vi "Encode (Single Param).vi"(9 "parameter in":dbl, 10 "parameter configuration":T1, 11 "words in":u16[](array[numeric]) format="%.0b") -> (3 "words out":u16[](array[numeric]) format="%.0b")   [LabVIEW 2020]
uses:
  _typedefs/parameter_config_type.ctl
  _typedefs/parameter_config_type_type.ctl
  _typedefs/parameter_config_encoding_type.ctl
  datatypes/dt_encodeDecode.lvlib
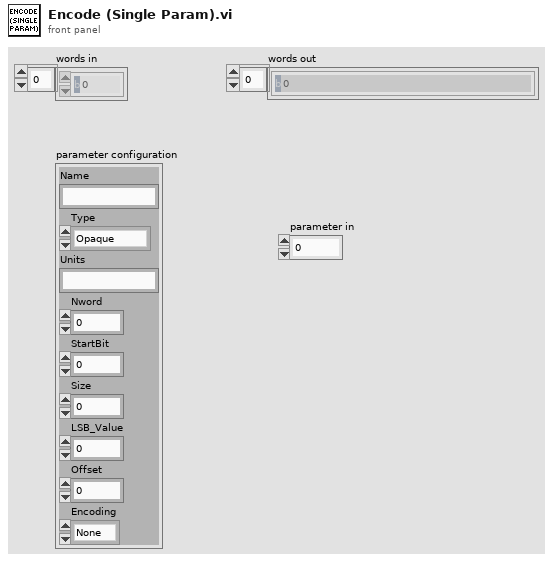
[diagram p1: front panel]
types:
  T1 = typedef "parameter_config_type.ctl" = cluster{"Name":string, "Type":T2, "Units":string, "Nword":i32, "StartBit":i32, "Size":i32, "LSB_Value":dbl, "Offset":i32, "Encoding":T3}
  T2 = typedef "parameter_config_type_type.ctl" = enum16{"Opaque", "Enum", "Float", "Integer", "Bcd", "Bool"}
  T3 = typedef "parameter_config_encoding_type.ctl" = enum16{"None", "2-complement", "Unsigned"}
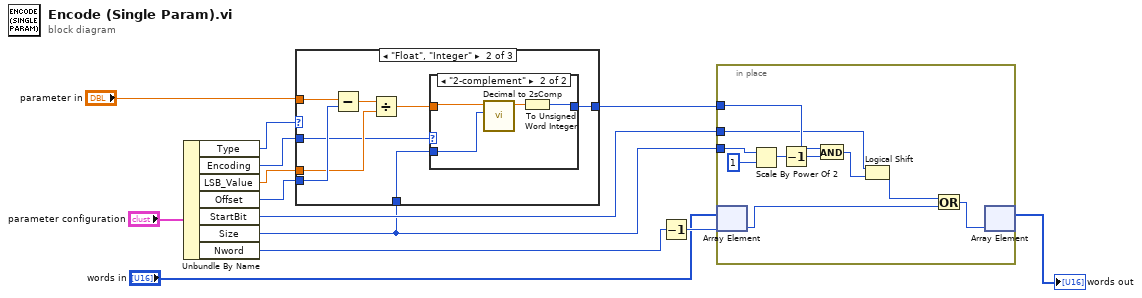
[diagram p0: block diagram]
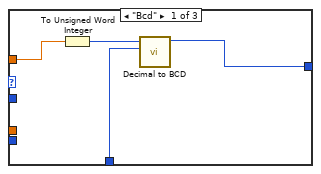
[diagram p2: hidden frame]
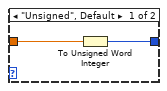
[diagram p3: hidden frame]
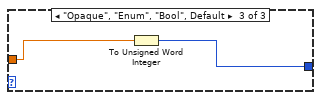
[diagram p4: hidden frame]
diagram:
  n1 = Unbundle By Name("parameter configuration") -> ("Type"=w6:T2, "Encoding"=w4:T3, "LSB_Value"=w3:dbl, "Offset"=w2:i32, "StartBit"=w12:i32, "Size"=w5:i32, "Nword"=w8:i32)
  n2 = case shown="\"Float\", \"Integer\"" w6 {
    tunnel: "parameter in" -> [w17 w25 w33]
    tunnel: w5 -> [w16 w18 _]
    tunnel: w4 -> [_ w21 _]
    tunnel: w3 -> [_ w22 _]
    tunnel: w2 -> [_ w24 _]
    tunnel: [w15 w19 w32] -> w1
    frame "Bcd" {
      n3 = To Unsigned Word Integer(number=w17) -> (unsigned 16bit integer=w14:u16)
      n4 = call "Decimal to BCD.vi"("size in bits"=w16, "decimal data in"=w14) -> ("bcd data out"=w15:u16)  [unwired: 9 in]
    }
    frame "Float", "Integer" {
      n5 = Subtract(x=w25, y=w24) -> (x-y=w23:dbl)
      n6 = Divide(x=w23, y=w22) -> (x/y=w20:dbl)
      n7 = case shown="\"2-complement\"" w21 {
        tunnel: w20 -> [w27 w30]
        tunnel: [w26 w28] -> w19
        tunnel: w18 -> [_ w31]
        frame "Unsigned", Default {
          n8 = To Unsigned Word Integer(number=w27) -> (unsigned 16bit integer=w26:u16)
        }
        frame "2-complement" {
          n9 = call "Decimal to 2sComp.vi"("size in bit"=w31, "decimal in"=w30) -> ("word out"=w29:dbl)  [unwired: 9 in]
          n10 = To Unsigned Word Integer(number=w29) -> (unsigned 16bit integer=w28:u16)
        }
      }
    }
    frame "Opaque", "Enum", "Bool", Default {
      n11 = To Unsigned Word Integer(number=w33) -> (unsigned 16bit integer=w32:u16)
    }
  }
  n12 = Decrement(x=w8) -> (x-1=w11:i32)
  n13 = in-place {
    in-place-border: w5 -> [w42]
    in-place-border: w1 -> [w39]
    in-place-border: w12 -> [w38]
    n14 = in-place-array #1("words in", w11) -> (w35:u16)
    n15 = Scale By Power Of 2(n=w42, x=u16 1) -> (x*2^n=w41:u16)
    n16 = Decrement(x=w41) -> (x-1=w40:u16)
    n17 = And(x=w39, y=w40) -> (x .and. y?=w37:u16)
    n18 = Logical Shift(y=w38, x=w37) -> (x << y=w36:u16)
    n19 = Or(x=w36, y=w35) -> (x .or. y?=w34:u16)
    n20 = in-place-array #1(w34) -> (→"words out":u16[])  [unwired: 1 out]
  }
